vi "Parameters_Get_Reference.vi"(8 "error in (no error)":errorcluster, 11 "Parameters":dbl[](array[numeric])) -> (0 "error out":errorcluster, 2 "Reference Move Parameters":T1={"Reference Move Mode"=3, "Start Search Forward"=FALSE, "Stop on FWD Edge"=FALSE, "Approach Forward"=FALSE, "Velocity"=0.0, "Acceleration"=0.0}, 3 "Axis to command":i32)   [LabVIEW 2017, in "WordManipulationLibrary.lvlib"]
uses:
  WordManipulationLibrary.lvlib
  Parameters_Reference.ctl
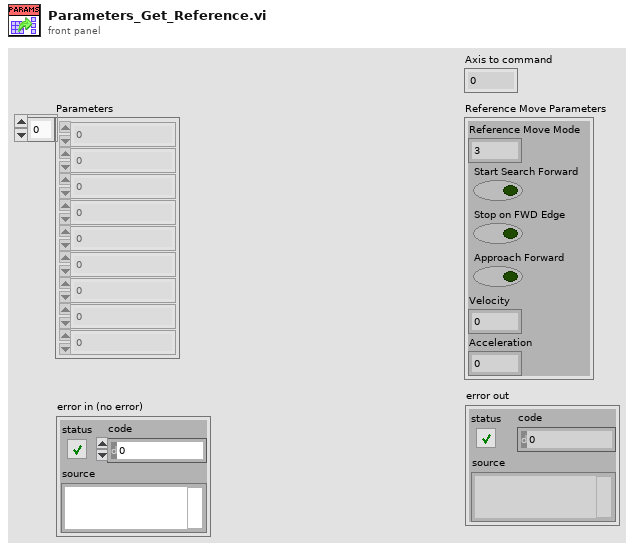
[diagram p1: front panel]
types:
  T1 = typedef "WordManipulationLibrary.lvlib/Parameters_Reference.ctl" = cluster{"Reference Move Mode":i32, "Start Search Forward":bool, "Stop on FWD Edge":bool, "Approach Forward":bool, "Velocity":dbl, "Acceleration":dbl}
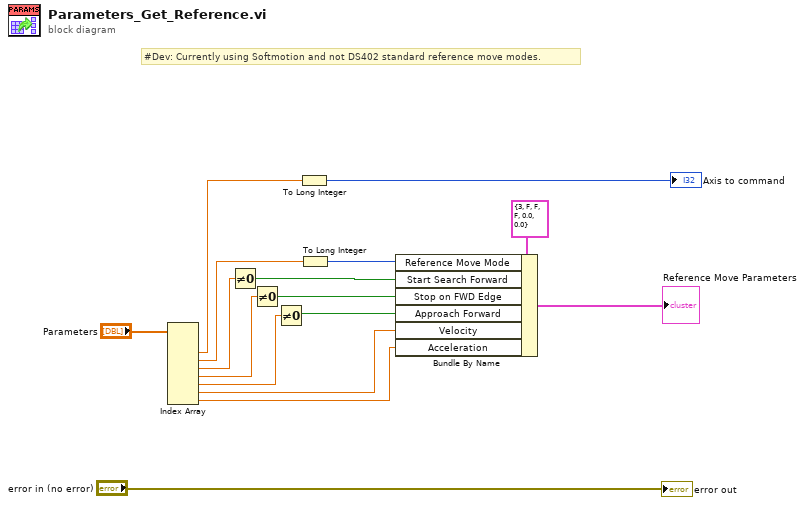
[diagram p0: block diagram]
diagram:
  # "#Dev: Currently using Softmotion and not DS402 standard reference move modes."
  n1 = Index Array(array="Parameters") -> (element #2=w2:dbl, element #3=w13:dbl, element #4=w9:dbl, element #5=w8:dbl, element #6=w7:dbl, element #7=w6:dbl, element #8=w10:dbl)  [unwired: 8 in, 1 out]
  n2 = Not Equal To 0?(x=w9) -> (x != 0?=w5:bool)
  n3 = Not Equal To 0?(x=w8) -> (x != 0?=w4:bool)
  n4 = Not Equal To 0?(x=w7) -> (x != 0?=w3:bool)
  n5 = To Long Integer(number=w2) -> (32bit integer=→"Axis to command":i32)
  n6 = To Long Integer(number=w13) -> (32bit integer=w14:i32)
  n7 = Bundle By Name(cluster=T1 {"Reference Move Mode"=3, "Start Search Forward"=FALSE, "Stop on FWD Edge"=FALSE, "Approach Forward"=FALSE, "Velocity"=0.0, "Acceleration"=0.0} ("output cluster 2"), "Reference Move Mode"=w14, "Start Search Forward"=w5, "Stop on FWD Edge"=w4, "Approach Forward"=w3, "Velocity"=w6, "Acceleration"=w10) -> (→"Reference Move Parameters":T1)
  "error out" <- "error in (no error)"
